vi "Write.vi"(7 "error in (no error)":errorcluster, 9 "Values":bool[](array[boolean]), 10 "DIO Ref In":T1) -> (0 "error out":errorcluster, 3 "DIO Ref Out":T1)   [LabVIEW 2021, in "DIO.lvlib"]
doc: "Writes logic levels to one or more digital I/O channels."
uses:
  <vilib>/myRIO/Instrument Drivers/Onboard IO/DIO/DIO.lvlib
  <vilib>/myRIO/Instrument Drivers/Onboard IO/DIO/typedefs/DIO Reference.ctl
  <vilib>/myRIO/Common/Instrument Driver Framework/Utilities/typedefs/myRIO Generic Hardware Reference.ctl
  <vilib>/myRIO/Common/Instrument Driver Framework/Utilities/typedefs/Hardware Version Enum.ctl
  <vilib>/myRIO/Common/Instrument Driver Framework/Utilities/typedefs/myRIO v1.0 Reference.ctl
  <vilib>/myRIO/Common/Instrument Driver Framework/Utilities/typedefs/Generic FPGA Reference.ctl
  <vilib>/myRIO/Common/Instrument Driver Framework/myRIO v1.0/DIO/typedefs/DIO Channels List.ctl
  <vilib>/myRIO/Common/Instrument Driver Framework/myRIO v1.0/DIO/typedefs/DIO Channels Enum.ctl
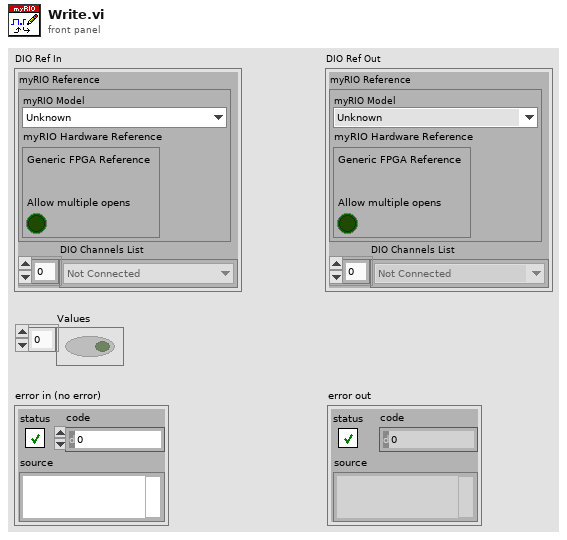
[diagram p1: front panel]
types:
  T1 = typedef "DIO.lvlib/DIO Reference.ctl" = cluster{"myRIO Reference":T2, "DIO Channels List":T6}
  T2 = typedef "myRIO Generic Hardware Reference.ctl" = cluster{"myRIO Model":T3, "myRIO Hardware Reference":T4}
  T3 = typedef "Hardware Version Enum.ctl" = enum16{"Unknown", "myRIO-1900", "myRIO-1950", "roboRIO", "NI ELVIS RIO CM", "ELVIS III"}
  T4 = typedef "myRIO v1.0 Reference.ctl" = cluster{"Generic FPGA Reference":T5, "Allow multiple opens":bool}
  T5 = typedef "Generic FPGA Reference.ctl" = refnum<k20>
  T6 = typedef "DIO Channels List.ctl" = T7[]
  T7 = typedef "DIO Channels Enum.ctl" = enum16{"Not Connected", "C/DIO0", "C/DIO1", "C/DIO2", "C/DIO3", "C/DIO4", "C/DIO5", "C/DIO6", "C/DIO7", "A/DIO0", "A/DIO1", "A/DIO2", "A/DIO3", "A/DIO4", "A/DIO5", "A/DIO6", "A/DIO7", "A/DIO8", "A/DIO9", "A/DIO10", "A/DIO11", "A/DIO12", "A/DIO13", "A/DIO14", "A/DIO15", "A/DIO16", "A/DIO17", "A/DIO18", "A/DIO19", "B/DIO0", "B/DIO1", "B/DIO2", "B/DIO3", "B/DIO4", "B/DIO5", "B/DIO6", "B/DIO7", "B/DIO8", "B/DIO9", "B/DIO10", "B/DIO11", "B/DIO12", "B/DIO13", "B/DIO14", "B/DIO15", "B/DIO16", "B/DIO17", "B/DIO18", "B/DIO19", "LED0", "LED1", "LED2", "LED3", "Button0", "DIO/DIO0", "DIO/DIO1", "DIO/DIO2", "DIO/DIO3", "DIO/DIO4", "DIO/DIO5", "DIO/DIO6", "DIO/DIO7", "DIO/DIO8", "DIO/DIO9", "SPI/CS0", "SPI/CS1", "SPI/CS2", "SPI/CS3", "LED RADIO (Green)", "LED RADIO (Red)", "LED COMM (Green)", "LED COMM (Red)", "LED MODE (Green)", "LED MODE (Red)"}
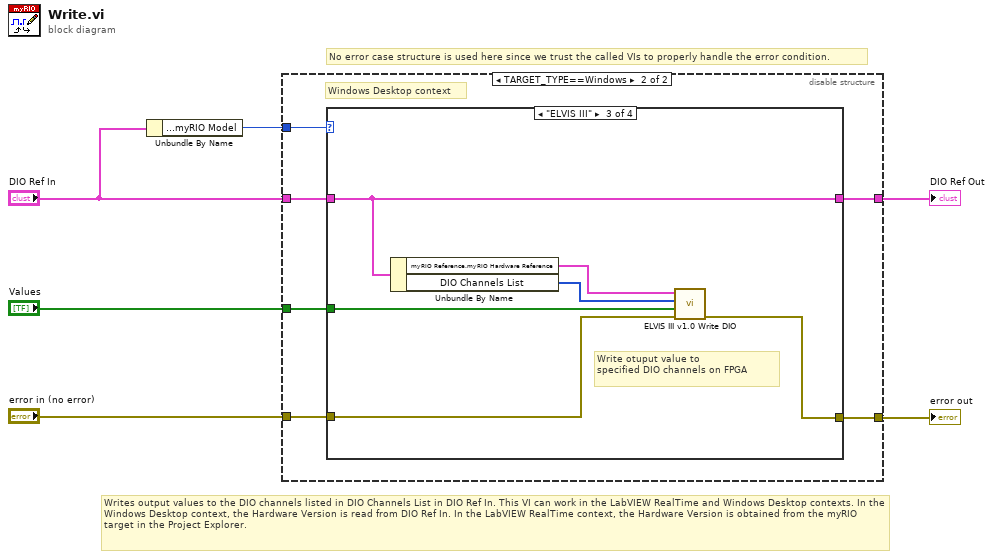
[diagram p0: block diagram]
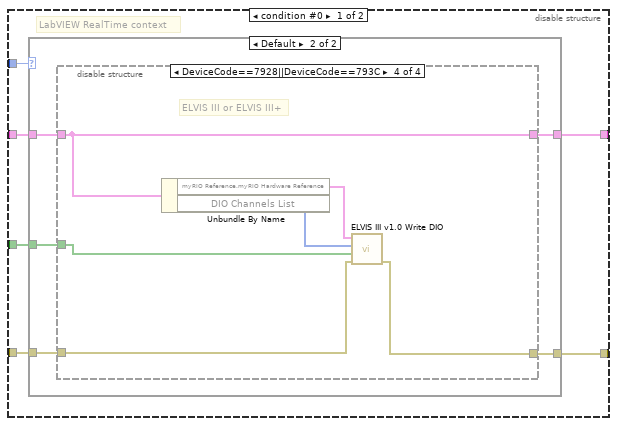
[diagram p2: hidden frame]
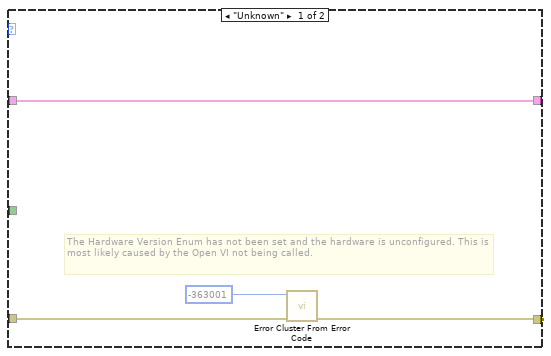
[diagram p3: hidden frame]
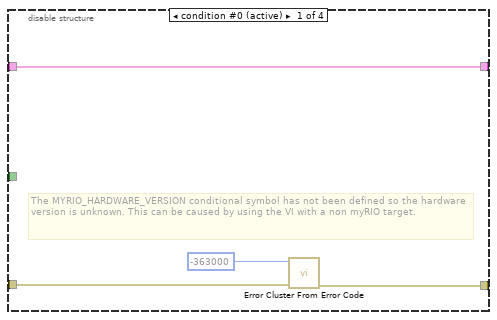
[diagram p4: hidden frame]
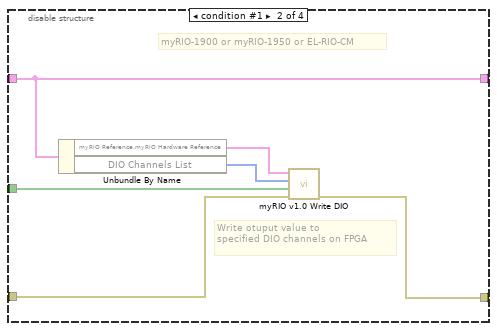
[diagram p5: hidden frame]
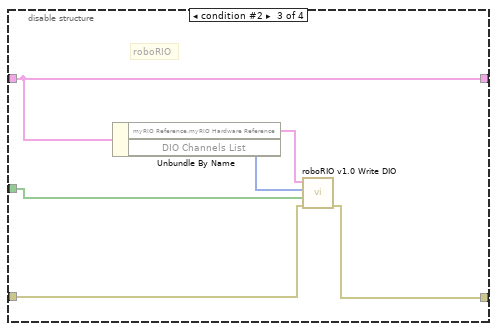
[diagram p6: hidden frame]
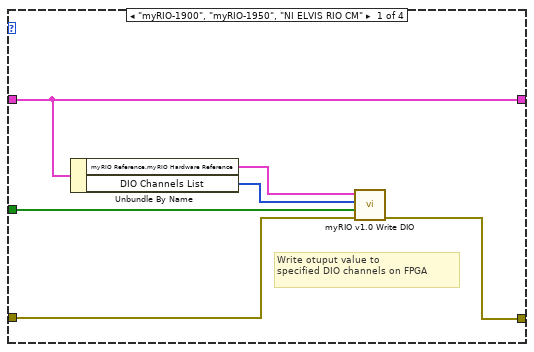
[diagram p7: hidden frame]
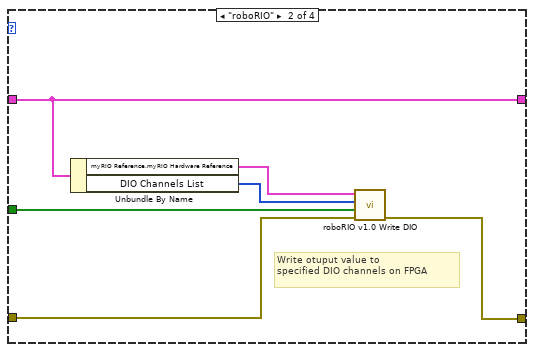
[diagram p8: hidden frame]
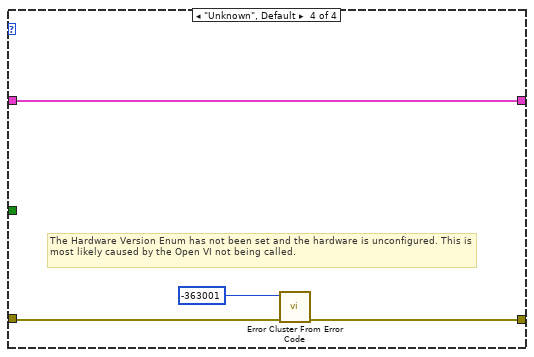
[diagram p9: hidden frame]
diagram:
  # "No error case structure is used here since we trust the called VIs to properly handle the error condition."
  # "Writes output values to the DIO channels listed in DIO Channels List in DIO Ref In. This VI can work in the LabVIEW RealTime and Windows Desktop contexts. In the Windows Desktop context, the Hardware Version is read from DIO Ref In. In the LabVIEW RealTime context, the Hardware Version is obtained from the myRIO target in the Project Explorer."
  n1 = Unbundle By Name("DIO Ref In") -> ("myRIO Reference.myRIO Model"=w1:T3)
  n2 = disable-structure shown="TARGET_TYPE==Windows" {
    disable-tunnel: [w12 w49] -> w3
    disable-tunnel: "DIO Ref In" -> [w11 w46]
    disable-tunnel: "error in (no error)" -> [w10 w48]
    disable-tunnel: [w9 w47] -> w4
    disable-tunnel: "Values" -> [w8 w45]
    disable-tunnel: w1 -> [w7 w44]
    frame condition #0 {
      # "LabVIEW RealTime context"
      n3 = case shown="Default" w7 {
        tunnel: [w15 w21] -> w12
        tunnel: w11 -> [w13 w20]
        tunnel: w10 -> [w14 w19]
        tunnel: [w13 w18] -> w9
        tunnel: w8 -> [_ w17]
        frame "Unknown" {
          # "The Hardware Version Enum has not been set and the hardware is unconfigured. This is most likely caused by the Open VI not being called."
          n4 = call <vilib>:"Error Cluster From Error Code.vi"("error in (no error)"=w14, "error code (0)"=-363001) -> ("error out"=w15:errorcluster)  [unwired: 7 in]
        }
        frame Default {
          n5 = disable-structure shown="DeviceCode==7928||DeviceCode==793C" {
            disable-tunnel: w20 -> [w22 w31 w37 w41]
            disable-tunnel: [w25 w28 w32 w40] -> w21
            disable-tunnel: w19 -> [w23 w30 w33 w39]
            disable-tunnel: [w22 w31 w37 w41] -> w18
            disable-tunnel: w17 -> [_ w27 w34 w38]
            frame condition #0 (active) {
              # "The MYRIO_HARDWARE_VERSION conditional symbol has not been defined so the hardware version is unknown. This can be caused by using the VI with a non myRIO target."
              n6 = call <vilib>:"Error Cluster From Error Code.vi"("error in (no error)"=w23, "error code (0)"=-363000) -> ("error out"=w25:errorcluster)  [unwired: 7 in]
            }
            frame condition #1 {
              # "myRIO-1900 or myRIO-1950 or EL-RIO-CM"
              # "Write otuput value to \nspecified DIO channels on FPGA"
              n7 = Unbundle By Name(w31) -> ("myRIO Reference.myRIO Hardware Reference"=w26:T4, "DIO Channels List"=w29:T6)
              n8 = call <vilib>:"myRIO v1.0 Write DIO.vi"("error in (no error)"=w30, "bool Value List"=w27, "Channel List"=w29, "myRIO Ref In"=w26) -> ("error out"=w28:errorcluster)  [unwired: 6 in, 1 out]
            }
            frame condition #2 {
              # "roboRIO"
              n9 = Unbundle By Name(w37) -> ("myRIO Reference.myRIO Hardware Reference"=w36:T4, "DIO Channels List"=w35:T6)
              n10 = call <vilib>:"roboRIO v1.0 Write DIO.vi"("error in (no error)"=w33, "bool Value List"=w34, "Channel List"=w35, "myRIO Ref In"=w36) -> ("error out"=w32:errorcluster)  [unwired: 6 in, 1 out]
            }
            frame condition #3 {
              # "ELVIS III or ELVIS III+"
              n11 = Unbundle By Name(w41) -> ("myRIO Reference.myRIO Hardware Reference"=w43:T4, "DIO Channels List"=w42:T6)
              n12 = call <vilib>:"ELVIS III v1.0 Write DIO.vi"("error in (no error)"=w39, "bool Value List"=w38, "Channel List"=w42, "myRIO Ref In"=w43) -> ("error out"=w40:errorcluster)  [unwired: 6 in, 1 out]
            }
          }
        }
      }
    }
    frame condition #1 (active) {
      # "Windows Desktop context"
      n13 = case shown="\"ELVIS III\"" w44 {
        tunnel: [w52 w58 w64 w71] -> w49
        tunnel: w46 -> [w55 w61 w65 w68]
        tunnel: w48 -> [w53 w59 w63 w69]
        tunnel: [w55 w61 w65 w68] -> w47
        tunnel: w45 -> [w51 w57 w62 _]
        frame "myRIO-1900", "myRIO-1950", "NI ELVIS RIO CM" {
          # "Write otuput value to \nspecified DIO channels on FPGA"
          n14 = Unbundle By Name(w55) -> ("myRIO Reference.myRIO Hardware Reference"=w50:T4, "DIO Channels List"=w54:T6)
          n15 = call <vilib>:"myRIO v1.0 Write DIO.vi"("error in (no error)"=w53, "bool Value List"=w51, "Channel List"=w54, "myRIO Ref In"=w50) -> ("error out"=w52:errorcluster)  [unwired: 6 in, 1 out]
        }
        frame "roboRIO" {
          # "Write otuput value to \nspecified DIO channels on FPGA"
          n16 = Unbundle By Name(w61) -> ("myRIO Reference.myRIO Hardware Reference"=w56:T4, "DIO Channels List"=w60:T6)
          n17 = call <vilib>:"roboRIO v1.0 Write DIO.vi"("error in (no error)"=w59, "bool Value List"=w57, "Channel List"=w60, "myRIO Ref In"=w56) -> ("error out"=w58:errorcluster)  [unwired: 6 in, 1 out]
        }
        frame "ELVIS III" {
          # "Write otuput value to \nspecified DIO channels on FPGA"
          n18 = Unbundle By Name(w65) -> ("myRIO Reference.myRIO Hardware Reference"=w66:T4, "DIO Channels List"=w67:T6)
          n19 = call <vilib>:"ELVIS III v1.0 Write DIO.vi"("error in (no error)"=w63, "bool Value List"=w62, "Channel List"=w67, "myRIO Ref In"=w66) -> ("error out"=w64:errorcluster)  [unwired: 6 in, 1 out]
        }
        frame "Unknown", Default {
          # "The Hardware Version Enum has not been set and the hardware is unconfigured. This is most likely caused by the Open VI not being called."
          n20 = call <vilib>:"Error Cluster From Error Code.vi"("error in (no error)"=w69, "error code (0)"=-363001) -> ("error out"=w71:errorcluster)  [unwired: 7 in]
        }
      }
    }
  }
  "DIO Ref Out" <- w4
  "error out" <- w3
